vi "Determine Packet Start.vi"(7 "samples to cut into cyclic prefix":u8, 8 "input valid":bool, 9 "last peak index":u16, 10 "number of consecutive peaks":u8) -> (0 "packet start valid":bool, 1 "STF start index after low pass filter":u16, 2 "L-LTF 2 start index":u16)   [LabVIEW 2020]
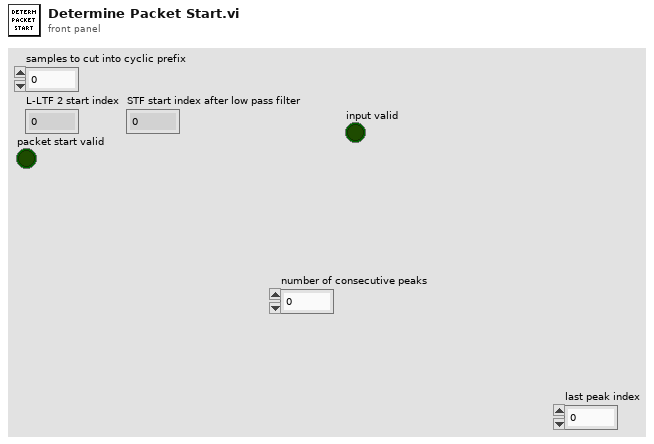
[diagram p1: front panel]
types:
  T1 = cluster{"EIFS":u32, "ACK timeout":u32, "CTS timeout":u32, "aRxPHYStartDelay":u32, "Frame control field length":u16, "Duration/ID field length":u16, "aSlotTime":u32, "aSIFSTime":u32, "PIFS":u32, "DIFS":u32, "Address field length":u16, "Sequence control field length":u16, "QoS control field length":u16, "HT control field length":u16, "FCS field length":u16, "MPDU delimiter length":u16, "MPDU delimiter signature":u16, "Max MPDU buffer length":u16, "timestamp steps / mks":u32, "L-STF periods / L-STF":u8, "sample / L-STF period":u8, "T_SIGNAL":u16, "N_tail":u16, "N_service":u16, "N_ES":u16, "N_SS":u16, "m_STBC":u16, "T_VHTSIGB":u16, "T_VHTPREAMBLE":u16, "T_VHTSIGA":u16, "T_LSIG":u16, "T_LEGPREAMBLE":u16, "NOFDM_VHTSIGB":u16, "T_SYM":u16, "T_SYML":u16, "NOFDM_PREAMBLE":u16, "NOFDM_SIGNAL":u16, "T_PREAMBLE":u16, "NOFDM_LEGPREAMBLE":u16, "NOFDM_VHTPREAMBLE":u16, "NOFDM_VHTSIGA":u16, "NOFDM_LSIG":u16, "NOFDM_VHTPREAMBLE 2":u16, "NOFDM_LSIG 2":u16}
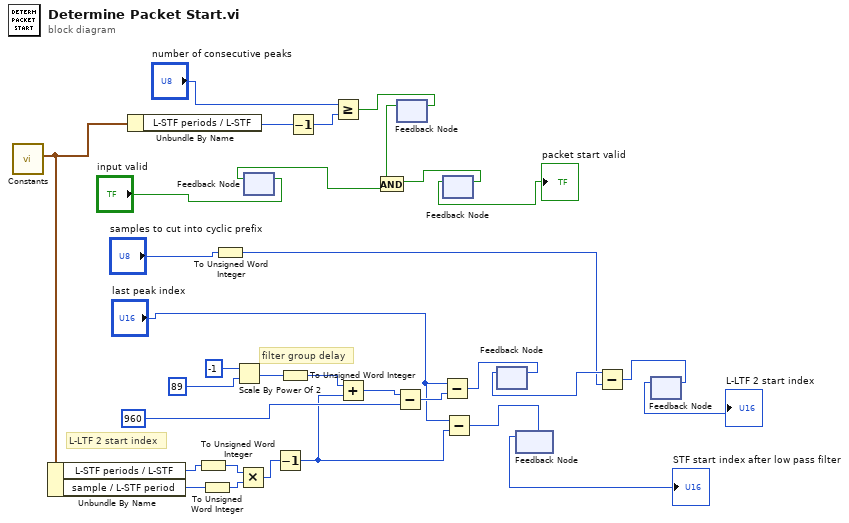
[diagram p0: block diagram]
diagram:
  # "filter group delay"
  # "L-LTF 2 start index"
  n1 = call "Constants.vi"() -> ("output cluster"=w9:T1)  [unwired: 11 in]
  n2 = Unbundle By Name(w9) -> ("L-STF periods / L-STF"=w14:u8, "sample / L-STF period"=w13:u8)
  n3 = Unbundle By Name(w9) -> ("L-STF periods / L-STF"=w32:u8)
  n4 = To Unsigned Word Integer(number=w14) -> (unsigned 16bit integer=w11:u16)
  n5 = To Unsigned Word Integer(number=w13) -> (unsigned 16bit integer=w12:u16)
  n6 = To Unsigned Word Integer(number="samples to cut into cyclic prefix") -> (unsigned 16bit integer=w4:u16)
  n7 = Scale By Power Of 2(n=i16 -1, x=u8 89 ("n")) -> (x*2^n=w21:u8)
  n8 = Multiply(x=w11, y=w12) -> (x*y=w10:u16)
  n9 = feedback #1() -> (w27:bool)  [unwired: 1 in]
  n10 = feedback-in #1("input valid") -> ()
  n11 = Decrement(x=w10) -> (x-1=w15:u16)
  n12 = To Unsigned Word Integer(number=w21) -> (unsigned 16bit integer=w20:u16)
  n13 = Decrement(x=w32) -> (x-1=w31:u8)
  n14 = Greater Or Equal?(x="number of consecutive peaks", y=w31) -> (x >= y?=w29:bool)
  n15 = Add(x=w20, y=w15) -> (x+y=w19:u16)
  n16 = Subtract(x=w19, y=u16 960) -> (x-y=w17:u16)
  n17 = feedback-in #2(w29) -> ()
  n18 = feedback #2() -> (w28:bool)  [unwired: 1 in]
  n19 = And(x=w28, y=w27) -> (x .and. y?=w25:bool)
  n20 = Subtract(x="last peak index", y=w17) -> (x-y=w7:u16)
  n21 = feedback #3() -> (→"packet start valid":bool)  [unwired: 1 in]
  n22 = feedback-in #3(w25) -> ()
  n23 = Subtract(x="last peak index", y=w15) -> (x-y=w8:u16)
  n24 = feedback #4() -> (w5:u16)  [unwired: 1 in]
  n25 = feedback-in #4(w7) -> ()
  n26 = feedback #5() -> (→"STF start index after low pass filter":u16)  [unwired: 1 in]
  n27 = feedback-in #5(w8) -> ()
  n28 = Subtract(x=w5, y=w4) -> (x-y=w3:u16)
  n29 = feedback #6() -> (→"L-LTF 2 start index":u16)  [unwired: 1 in]
  n30 = feedback-in #6(w3) -> ()
